vi "Example Callback.vi"() -> ()   [LabVIEW 2013]
uses:
  C:/tf/play/labview/Tinkerforge.dll
  Tinkerforge.dll
panel:
  out "pm10.0 (µg/m³)":u16
  out "pm2.5 (µg/m³)":u16
  out "pm1.0 (µg/m³)":u16
  in  "stop":bool
  in  "uid":string="abc"
  in  "port":i32=4223
  in  "host":string="localhost"
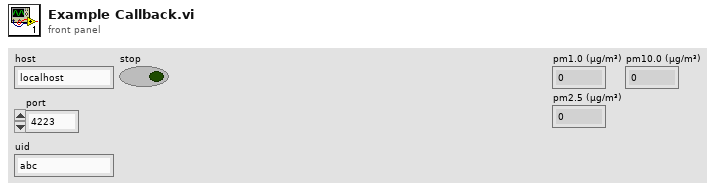
[diagram p1: front panel]
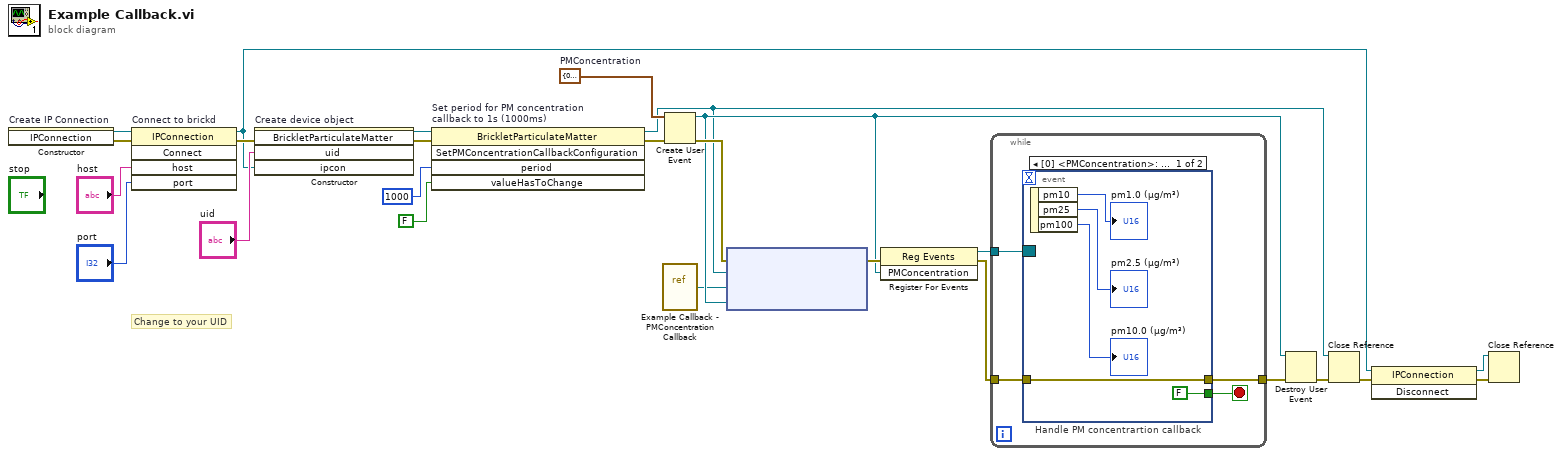
[diagram p0: block diagram]
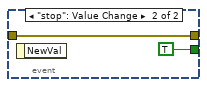
[diagram p2: hidden frame]
diagram:
  w9 = cluster{"pm10":i32, "pm25":i32, "pm100":i32} {"pm10"=0, "pm25"=0, "pm100"=0}  # PMConcentration
  # "Change to your UID"
  n1 = constructor on="Create IP Connection" class="IPConnection"() -> (reference out=w25:refnum<k24>, error out=w3:errorcluster)  [unwired: 3 in, 1 out]
  n2 = invoke on="Connect to brickd" class="IPConnection" method="Connect"(reference=w25, error in=w3, "host"="host", "port"="port") -> (reference out=w18:refnum<k24>, error out=w21:errorcluster)  [unwired: 1 in, 3 out]
  n3 = constructor on="Create device object" class="BrickletParticulateMatter"(error in=w21, "uid"="uid", "ipcon"=w18) -> (reference out=w6:refnum<k24>, error out=w8:errorcluster)  [unwired: 2 in, 3 out]
  n4 = invoke on="Set period for PM concentration\ncallback to 1s (1000ms)" class="BrickletParticulateMatter" method="SetPMConcentrationCallbackConfiguration"(reference=w6, error in=w8, "period"=i64 1000, "valueHasToChange"=FALSE) -> (reference out=w5:refnum<k24>, error out=w7:errorcluster)  [unwired: 1 in, 3 out]
  n5 = vi-ref "Example Callback - PMConcentration Callback.vi"() -> ("vi reference"=w1:refnum<vi>)
  n6 = Create User Event(user event datatype=w9, error in=w7) -> (user event=w11:refnum<user-event>, error out=w16:errorcluster)
  n7 = node ("Register Event Callback")(w16, w5, w1, w11) -> (w15:errorcluster)  [unwired: 1 in, 1 out]
  n8 = register-events(error in=w15, w11) -> (reference out=w14:refnum<event-registration>, error out=w12:errorcluster)  [unwired: 1 in]
  n9 = while {
    tunnel: w14 -> [w29]
    tunnel: [w28] -> w13
    tunnel: w12 -> [w27]
    stop <- w26 stop-if-true
    n10 = event "Handle PM concentrartion callback" shown="[0] <PMConcentration>: User Event" {
      selector: w29 -> [_ _]
      dyn-events: _ -> [_ _]
      timeout: _ -> [_ _]
      tunnel: [w34 w35] -> w28
      tunnel: w27 -> [w34 w35]
      tunnel: [FALSE TRUE] -> w26
      event User Event {
        n11 = event-data() -> ("pm10"=→"pm1.0 (µg/m³)":i32, "pm25"=→"pm2.5 (µg/m³)":i32, "pm100"=→"pm10.0 (µg/m³)":i32)  [unwired: 1 in]
      }
      event "stop": Value Change {
        n12 = event-data() -> ()  [unwired: 1 in, 1 out]
      }
    }
  }
  n13 = Destroy User Event(user event=w11, error in=w13) -> (error out=w10:errorcluster)
  n14 = Close Reference(reference=w5, error in (no error)=w10) -> (error out=w20:errorcluster)
  n15 = invoke class="IPConnection" method="Disconnect"(reference=w18, error in=w20) -> (reference out=w17:refnum<k24>, error out=w19:errorcluster)  [unwired: 1 in, 1 out]
  n16 = Close Reference(reference=w17, error in (no error)=w19) -> ()  [unwired: 1 out]
